vi "Inverse Kinematics.vi"(5 "leg":dbl caption="leg lenght", 6 "h":dbl caption="Platform Height", 7 "crank":dbl caption="crank lenght", 8 "B":dbl caption="Base R", 9 "P":dbl caption="Platfomr R", 10 "Heave":dbl, 11 "R":cluster{"x":dbl, "y":dbl, "z":dbl} caption="Rotations") -> (3 "motor":cluster{dbl, dbl, dbl})   [LabVIEW 2019]
uses:
  <vilib>/Analysis/baseanly.llb/Real A x B.vi
  <vilib>/Analysis/Matrix/Numeric/Add/Add - RM,RM.vi
  <vilib>/Analysis/Matrix/Numeric/Subtract/Subtract - RM,RM.vi
  <vilib>/Analysis/NI_AALBase.lvlib
  <vilib>/Analysis/Matrix/NI_Matrix.lvlib
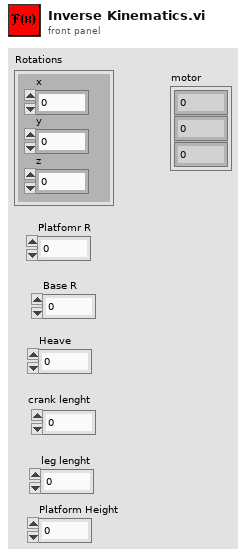
[diagram p1: front panel]
types:
  T1 = typedef "NI_Matrix.lvlib/RealMatrix.ctl" = dbl[][]
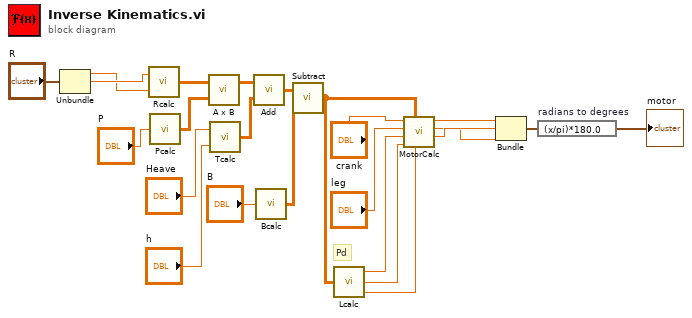
[diagram p0: block diagram]
diagram:
  # "Pd"
  n1 = Unbundle("R") -> ("x"=w3:dbl, "y"=w4:dbl)  [unwired: 1 out]
  n2 = call "Rcalc.vi"("roll"=w3, "pitch"=w4) -> ("appended array"=w19:T1)
  n3 = call "Pcalc.vi"("patR"="P") -> ("P"=w18:T1)
  n4 = call-poly <vilib>:"A x B.vi"("B"=w18, "A"=w19) -> ("A x B"=w17:T1)  [unwired: 1 out]
  n5 = call "Tcalc.vi"("height"="h", "heave"="Heave") -> ("appended array"=w16:T1)
  n6 = call-poly <vilib>:"Add.vi"("Real Matrix B"=w16, "Real Matrix A"=w17) -> ("A + B"=w15:T1)
  n7 = call "Bcalc.vi"("baseR"="B") -> ("B"=w14:T1)
  n8 = call-poly <vilib>:"Subtract.vi"("Real Matrix B"=w14, "Real Matrix A"=w15) -> ("A - B"=w11:T1)
  n9 = call "Lcalc.vi"("A - B"=w11) -> ("l3"=w8:dbl, "l2"=w9:dbl, "l1"=w10:dbl)  [unwired: 2 in]
  n10 = call "MotorCalc.vi"("l3"=w8, "Pd"=w11, "l2"=w9, "l1"=w10, "leg"="leg", "crank"="crank") -> ("m3"=w2:dbl, "m2"=w1:dbl, "m1"=w6:dbl)  [unwired: 3 in]
  n11 = Bundle("m1"=w6, "m3"=w2, "m2"=w1) -> (w5:cluster{"m1":dbl, "m3":dbl, "m2":dbl})  [unwired: 1 in]
  n12 = expression code="(x/pi)*180.0" "radians to degrees"(w5) -> (→"motor":cluster{"m1":dbl, "m3":dbl, "m2":dbl})
